vi "OpenCommunications .vi"(8 "error in (no error)":errorcluster, 11 "StepMotor in":refnum<class "StepMotor.lvclass">) -> (0 "error out":errorcluster, 3 "StepMotor out":refnum<class "StepMotor.lvclass">)   [LabVIEW 2010, in "StepMotor.lvclass"]
doc: "Открытие соединения с привода СПШ"
uses:
  StepMotor.lvclass
  StepMotor.lvclass/StepMotor.ctl
  <vilib>/Instr/_visa.llb/VISA Configure Serial Port (Instr).vi
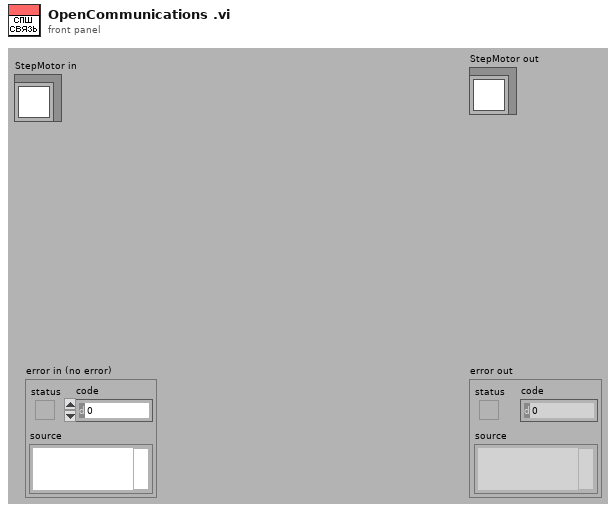
[diagram p1: front panel]
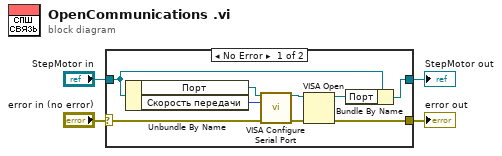
[diagram p0: block diagram]
diagram:
  n1 = case shown="No Error" "error in (no error)" {
    selector: "error in (no error)" -> [w5 w15]
    tunnel: [w12 w15] -> w3
    tunnel: [w10 w14] -> w2
    tunnel: "StepMotor in" -> [w11 w14]
    frame No Error {
      n2 = Unbundle By Name(w11) -> ("Порт"=w9:refnum<visa-resource-name>, "Скорость передачи"=w8:u32)
      n3 = call-poly "VISA Configure Serial Port"("VISA resource name"=w9, "baud rate (9600)"=w8, "error in (no error)"=w5) -> ("VISA resource name out"=w7:refnum<visa-resource-name>, "error out"=w6:errorcluster)  [unwired: 11 in]
      n4 = VISA Open(error in (no error)=w6, VISA resource name=w7) -> (VISA resource name=w13:refnum<visa-resource-name>, error out=w12:errorcluster)  [unwired: 3 in]
      n5 = Bundle By Name(cluster=w11, "Порт"=w13) -> (w10:refnum<class "StepMotor.lvclass">)
    }
    frame Error {
    }
  }
  "error out" <- w3
  "StepMotor out" <- w2
